vi "Lowspeed Mode.vi"(0 "section":string, 4 "Time Parameter":T1 {"Clock Frequency" format="%#_g KHz"; "T hd:sta" format="%#_g µs"; "T low" format="%#_g µs"; "T high" format="%#_g µs"; "T su:sta" format="%#_g µs"; "T hd:dat" format="%#_g µs"; "T su:dat" format="%#_g ns"; "T su:sto" format="%#_g µs"; "T buf" format="%#_g µs"}, 5 "DVR":refnum<data-value>, 11 "error in":errorcluster) -> (6 "This VI":refnum<vi>, 15 "error out":errorcluster)   [LabVIEW 2020, in "Low Speed.lvclass"]
uses:
  Low Speed.lvclass
  Parent Class/Speed Mode/Speed Mode.lvclass
  Typedefs/User event operator.ctl
  <vilib>/Utility/config.llb/Read Key (Double).vi
  I2C Controller.lvlib
  <vilib>/Utility/config.llb/NI_LVConfig.lvlib
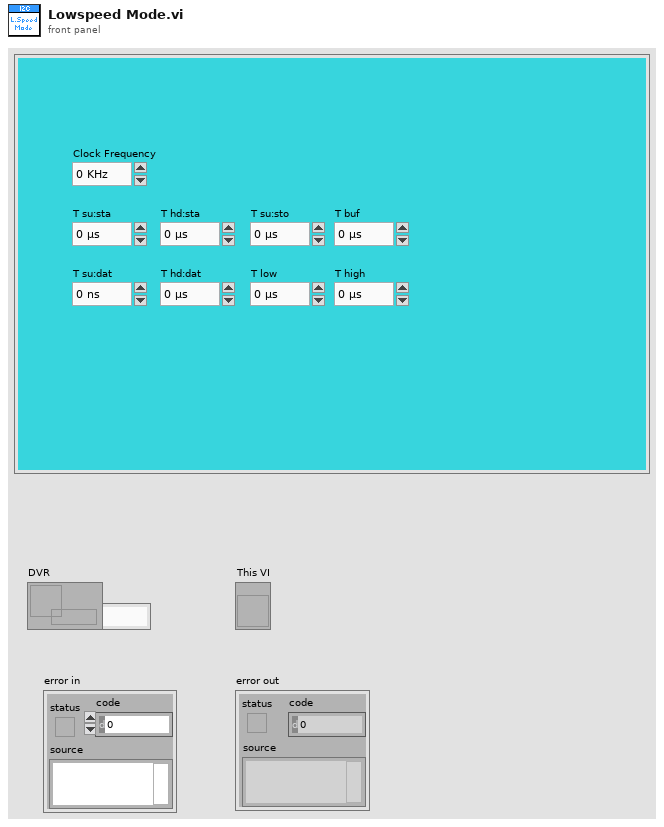
[diagram p1: front panel]
types:
  T1 = cluster{"Clock Frequency":dbl, "T hd:sta":dbl, "T low":dbl, "T high":dbl, "T su:sta":dbl, "T hd:dat":dbl, "T su:dat":dbl, "T su:sto":dbl, "T buf":dbl}
  T2 = typedef "I2C Controller.lvlib/User event operator.ctl" = enum16{"Create", "Generate Stop", "Destroy"}
  T3 = typedef "NI_LVConfig.lvlib/Config Data RefNum.ctl" = refnum<k1>
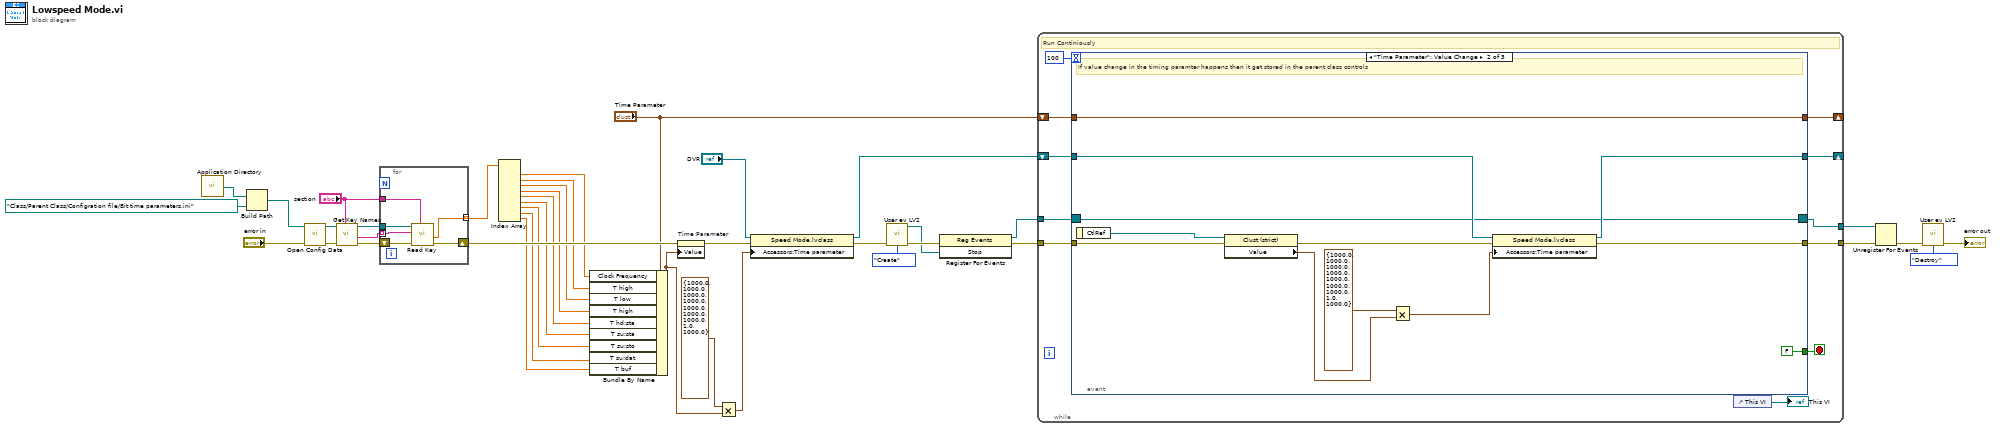
[diagram p0: block diagram]
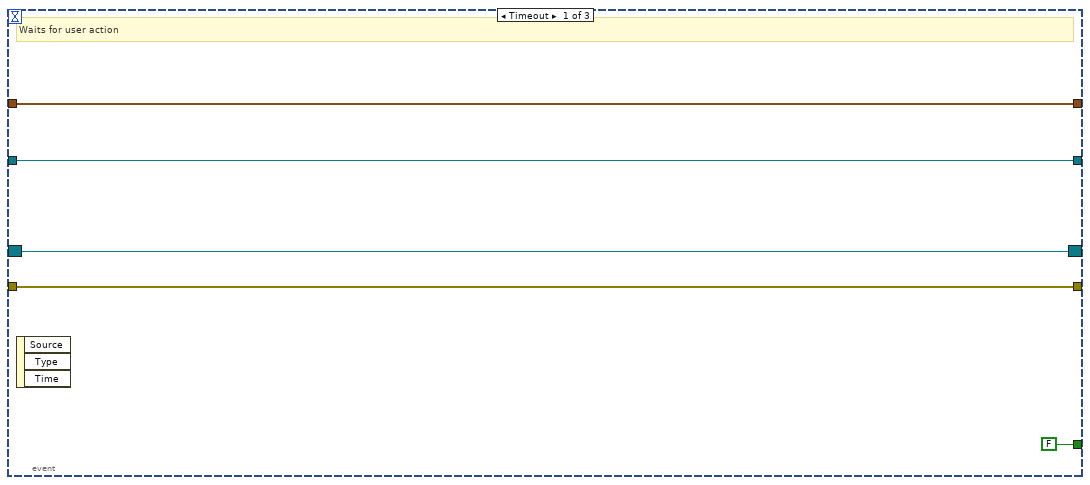
[diagram p2: hidden frame]
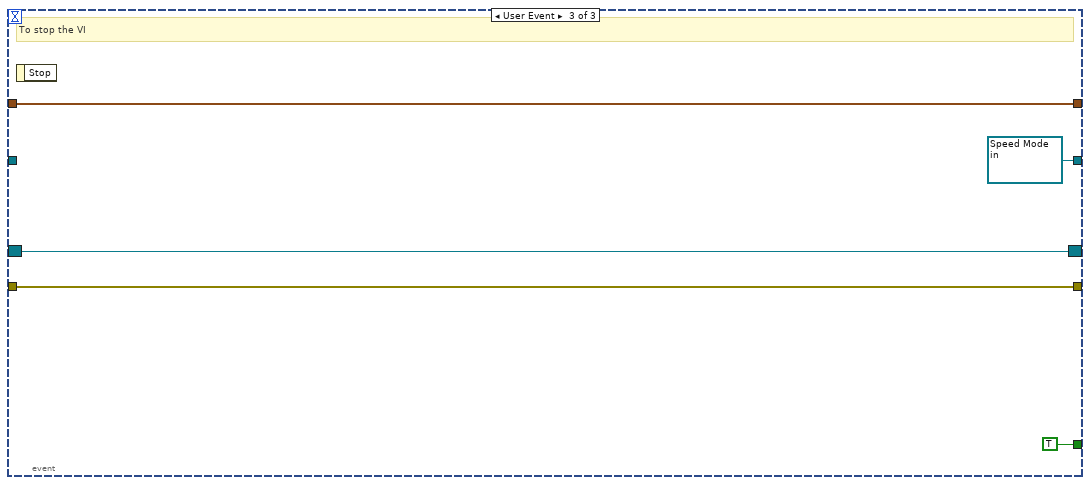
[diagram p3: hidden frame]
diagram:
  n1 = call <vilib>:"Application Directory.vi"() -> ("Application Directory"=w26:path)
  n2 = Build Path(base path=w26, name or relative path=path "Class/Parent Class/Configration file/Bit time parameters.ini") -> (appended path=w24:path)
  n3 = call <vilib>:"Open Config Data.vi"("error in (no error)"="error in", "configuration file path"=w24) -> ("error out"=w27:errorcluster, "refnum"=w23:T3)  [unwired: 7 in, 1 out]
  n4 = call <vilib>:"Get Key Names.vi"("section"="section", "error in (no error)"=w27, "refnum"=w23) -> ("error out"=w28:errorcluster, "key names"=w21:string[], "refnum out"=w22:T3)  [unwired: 5 in, 1 out]
  n5 = for {
    tunnel: "section" -> [w41]
    shift-right: [w44] -> w29
    shift-left: w28 -> [w45]
    tunnel: [w43] -> w20 mode=indexing
    tunnel: w22 -> [w42]
    tunnel: w21 -> [w40] mode=indexing
    n6 = call-poly <vilib>:"Read Key.vi"("section"=w41, "error in (no error)"=w45, "key"=w40, "refnum"=w42) -> ("error out"=w44:errorcluster, "value"=w43:dbl)  [unwired: 4 in, 2 out]
  }
  n7 = Index Array(array=w20) -> (element #1=w18:dbl, element #2=w17:dbl, element #3=w16:dbl, element #4=w15:dbl, element #5=w14:dbl, element #6=w13:dbl, element #7=w12:dbl, element #8=w11:dbl, element #9=w10:dbl)  [unwired: 9 in]
  n8 = Bundle By Name(cluster="Time Parameter", "Clock Frequency"=w18, "T high"=w17, "T low"=w16, "T high"=w15, "T hd:sta"=w14, "T su:sta"=w13, "T su:sto"=w12, "T su:dat"=w11, "T buf"=w10) -> (w3:T1)
  n9 = property on="Time Parameter" class="Clust (strict)"(error in=w29, "Value"=w3) -> (error out=w8:errorcluster)  [unwired: 1 in, 1 out]
  n10 = Multiply(x=T1 {"Clock Frequency"=1000.0, "T hd:sta"=1000.0, "T low"=1000.0, "T high"=1000.0, "T su:sta"=1000.0, "T hd:dat"=1000.0, "T su:dat"=1000.0, "T su:sto"=1.0, "T buf"=1000.0}, y=w3) -> (x*y=w1:T1)
  n11 = property class="Speed Mode.lvclass"(reference="DVR", error in=w8, "Accessors:Time parameter"=w1) -> (reference out=w5:refnum<data-value>, error out=w7:errorcluster)
  n12 = call "User ev LV2.vi"("Error in"=w7, "User Event Operator"=User_event_operator."Create") -> ("Stop"=w4:refnum<user-event>, "Error out"=w37:errorcluster)  [unwired: 12 in]
  n13 = register-events(error in=w37, w4) -> (reference out=w35:refnum<event-registration>, error out=w38:errorcluster)  [unwired: 1 in]
  n14 = while {
    tunnel: [w56] -> w39
    shift-right: [w53] -> _
    shift-left: "Time Parameter" -> [w52]
    tunnel: w38 -> [w51]
    tunnel: w35 -> [w50]
    shift-right: [w49] -> _
    shift-left: w5 -> [w47]
    tunnel: [w48] -> w33
    stop <- w46 stop-if-true
    # "Run Continiously"
    n15 = event shown="[1] \"Time Parameter\": Value Change" {
      selector: w50 -> [w57 w66 w77]
      dyn-events: [w57 w66 w77] -> w48
      timeout: 100 -> [_ _ _]
      tunnel: w52 -> [w61 w70 w75]
      tunnel: [w60 w71 w76] -> w56
      tunnel: [w61 w70 w75] -> w53
      tunnel: w51 -> [w60 w69 w76]
      tunnel: [w58 w67 refnum<data-value> refnum ("DVR")] -> w49
      tunnel: w47 -> [w58 w68 _]
      tunnel: [FALSE FALSE TRUE] -> w46
      event Timeout {
        # "Waits for user action"
        n16 = event-data() -> ()  [unwired: 1 in, 3 out]
      }
      event "Time Parameter": Value Change {
        # "If value change in the timing paramter happens then it get stored in the parent class controls"
        n17 = event-data() -> ("CtlRef"=w73:refnum<vi>)  [unwired: 1 in]
        n18 = property class="Clust (strict)"(reference=w73, error in=w69) -> (error out=w72:errorcluster, "Value"=w63:T1)  [unwired: 1 out]
        n19 = Multiply(x=T1 {"Clock Frequency"=1000.0, "T hd:sta"=1000.0, "T low"=1000.0, "T high"=1000.0, "T su:sta"=1000.0, "T hd:dat"=1000.0, "T su:dat"=1000.0, "T su:sto"=1.0, "T buf"=1000.0}, y=w63) -> (x*y=w62:T1)
        n20 = property class="Speed Mode.lvclass"(reference=w68, error in=w72, "Accessors:Time parameter"=w62) -> (reference out=w67:refnum<data-value>, error out=w71:errorcluster)
      }
      event User Event {
        # "To stop the VI"
        n21 = event-data() -> ()  [unwired: 1 in, 1 out]
      }
    }
    n22 = control-ref of="This VI"() -> (→"This VI":refnum<vi>)
  }
  n23 = Unregister For Events(event registration refnum=w33, error in=w39) -> (error out=w34:errorcluster)
  n24 = call "User ev LV2.vi"("Error in"=w34, "User Event Operator"=User_event_operator."Destroy") -> ("Error out"=→"error out":errorcluster)  [unwired: 12 in, 1 out]
